vi "15_2b.vi"() -> ()   [LabVIEW 2018]
panel:
  in  "Turn":i32=2020
  out "element":u64=232
  in  "Input":string="2,1,10,11,0,6"
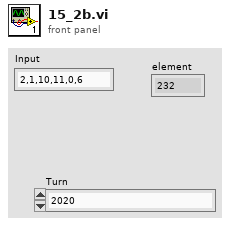
[diagram p1: front panel]
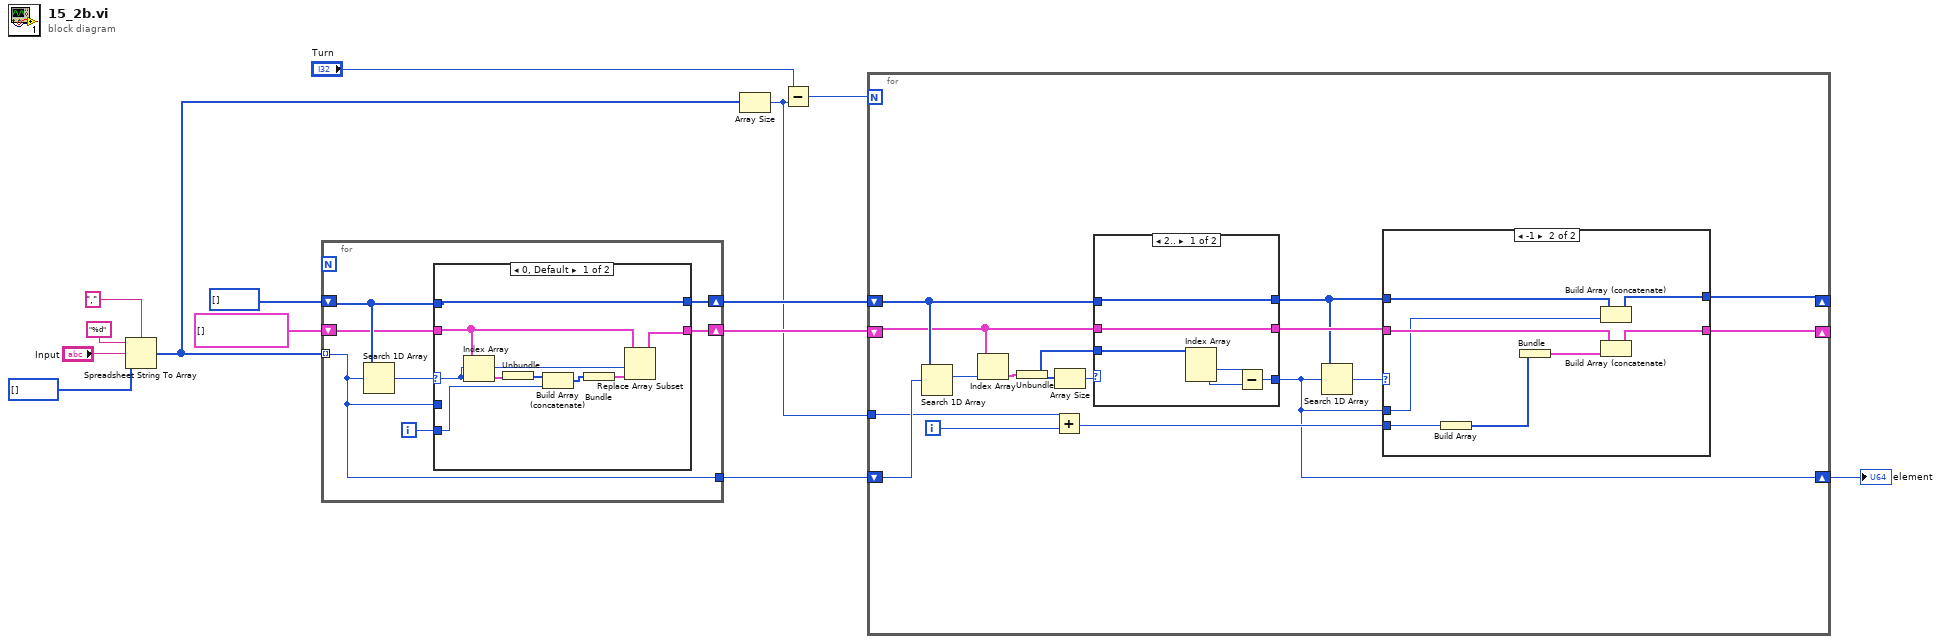
[diagram p0: block diagram]
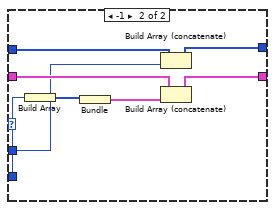
[diagram p2: hidden frame]
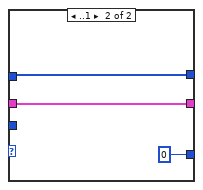
[diagram p3: hidden frame]
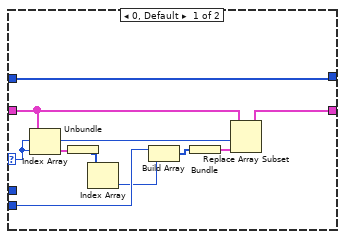
[diagram p4: hidden frame]
diagram:
  n1 = Spreadsheet String To Array(delimiter (Tab)=",", format string="%d", spreadsheet string="Input", array type (2D Dbl)=u64[] []) -> (array=w8:u64[])
  n2 = for {
    tunnel: w8 -> [w15] mode=indexing
    shift-right: [w19] -> w5
    shift-left: i32[] [] -> [w20]
    shift-right: [w16] -> w2
    shift-left: cluster{i32[]}[] [] -> [w18]
    tunnel: [w15] -> w4
    i -> [w17]
    n3 = Search 1D Array(1D array=w20, element=w15) -> (index of element=w21:i32)  [unwired: 1 in]
    n4 = case shown="0, Default" w21 {
      selector: w21 -> [w25 _]
      tunnel: w20 -> [w30 w38]
      tunnel: [w30 w37] -> w19
      tunnel: w18 -> [w24 w36]
      tunnel: w17 -> [w26 w32]
      tunnel: [w22 w33] -> w16
      tunnel: w15 -> [_ w31]
      frame 0, Default {
        n5 = Index Array(array=w24, index=w25) -> (element=w29:cluster{i32[]})
        n6 = Unbundle(w29) -> (w28:i32[])
        n7 = Build Array (concatenate)(w28, w26) -> (w27:i32[])
        n8 = Bundle(w27) -> (w23:cluster{i32[]})  [unwired: 1 in]
        n9 = Replace Array Subset(array=w24, new element=w23, index=w25) -> (w22:cluster{i32[]}[])
      }
      frame -1 {
        n10 = Build Array(w32) -> (w35:i32[])
        n11 = Bundle(w35) -> (w34:cluster{i32[]})  [unwired: 1 in]
        n12 = Build Array (concatenate)(w38, w31) -> (w37:u64[])
        n13 = Build Array (concatenate)(w36, w34) -> (w33:cluster{i32[]}[])
      }
    }
  }
  n14 = Array Size(array=w8) -> (size(s)=w1:i32)
  n15 = Subtract(x="Turn", y=w1) -> (x-y=w9:i32)
  n16 = for {
    N: w9 -> [_]
    shift-right: [w42] -> _
    shift-left: w5 -> [w53]
    shift-right: [w39] -> w3
    shift-left: w4 -> [w54]
    shift-right: [w41] -> _
    shift-left: w2 -> [w49]
    tunnel: w1 -> [w51]
    i -> [w52]
    n17 = Search 1D Array(1D array=w53, element=w54) -> (index of element=w48:i32)  [unwired: 1 in]
    n18 = Index Array(array=w49, index=w48) -> (element=w50:cluster{i32[]})
    n19 = Unbundle(w50) -> (w46:i32[])
    n20 = Add(x=w51, y=w52) -> (x+y=w40:i32)
    n21 = Array Size(array=w46) -> (size(s)=w47:i32)
    n22 = case shown="2.." w47 {
      tunnel: w53 -> [w58 w61]
      tunnel: [w58 w61] -> w43
      tunnel: w49 -> [w59 w62]
      tunnel: [w59 w62] -> w44
      tunnel: w46 -> [w57 _]
      tunnel: [w60 0] -> w39
      frame 2.. {
        n23 = Index Array(array=w57) -> (element #1=w56:i32, element #2=w55:i32)  [unwired: 2 in]
        n24 = Subtract(x=w56, y=w55) -> (x-y=w60:i32)
      }
      frame ..1 {
      }
    }
    n25 = Search 1D Array(1D array=w43, element=w39) -> (index of element=w45:i32)  [unwired: 1 in]
    n26 = case shown="-1" w45 {
      selector: w45 -> [w67 _]
      tunnel: [w69 w81] -> w42
      tunnel: w44 -> [w70 w80]
      tunnel: [w68 w78] -> w41
      tunnel: w43 -> [w69 w77]
      tunnel: w40 -> [w65 w76]
      tunnel: w39 -> [_ w74]
      frame 0, Default {
        n27 = Index Array(array=w70, index=w67) -> (element=w71:cluster{i32[]})
        n28 = Unbundle(w71) -> (w66:i32[])
        n29 = Index Array(array=w66) -> (element=w64:i32)  [unwired: 1 in]
        n30 = Build Array(w65, w64) -> (w72:i32[])
        n31 = Bundle(w72) -> (w73:cluster{i32[]})  [unwired: 1 in]
        n32 = Replace Array Subset(array=w70, new element=w73, index=w67) -> (w68:cluster{i32[]}[])
      }
      frame -1 {
        n33 = Build Array(w76) -> (w75:i32[])
        n34 = Bundle(w75) -> (w79:cluster{i32[]})  [unwired: 1 in]
        n35 = Build Array (concatenate)(w77, w74) -> (w81:u64[])
        n36 = Build Array (concatenate)(w80, w79) -> (w78:cluster{i32[]}[])
      }
    }
  }
  "element" <- w3
